vi "GetVIReference.vi"(5 "LVClassLibrary in":refnum<vi>, 6 "template (if new)":path, 7 "application reference":refnum<vi>, 8 "error in":errorcluster, 9 "not in class":bool, 10 "vi type":T1(ring), 11 "file path":path) -> (0 "error out":errorcluster, 3 "reference out":refnum<vi>)   [LabVIEW 2013, in "control module data interface generator.lvlib"]
doc: "This VI creates a new file or open the reference if the file already exists"
uses:
  control module data interface generator.lvlib
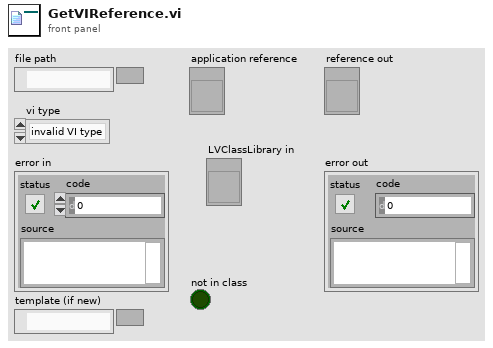
[diagram p1: front panel]
types:
  T1 = enum32{"invalid VI type", "Standard VI", "Control VI", "Global VI", "Polymorphic VI", "Configuration VI", "SubSystem", "Facade VI", "Method VI"}
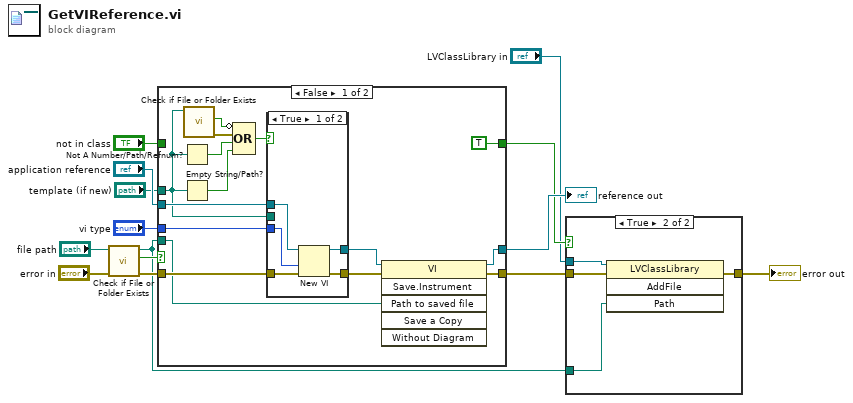
[diagram p0: block diagram]
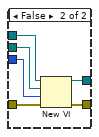
[diagram p3: hidden frame]
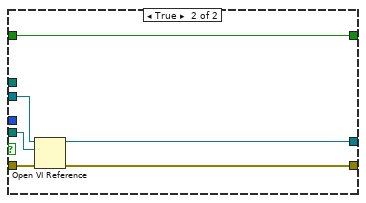
[diagram p4: hidden frame]
diagram:
  n1 = call <vilib>:"Check if File or Folder Exists.vi"("error in (no error)"="error in", "path"="file path") -> ("error out"=w12:errorcluster, "file or folder exists?"=w13:bool, "dup path"=w4:path)  [unwired: 7 in]
  n2 = case shown="False" w13 {
    tunnel: [w24 w44] -> w9
    tunnel: w12 -> [w29 w45]
    tunnel: w4 -> [w23 w46]
    tunnel: [w22 w43] -> w6
    tunnel: "vi type" -> [w27 _]
    tunnel: "application reference" -> [w26 w42]
    tunnel: [TRUE ("not in class") w41] -> w3
    tunnel: "not in class" -> [_ w41]
    tunnel: "template (if new)" -> [w16 _]
    frame False {
      n3 = Not A Number/Path/Refnum?(number/path/refnum=w16) -> (NaN/Path/Refnum?=w17:bool)
      n4 = Empty String/Path?(string/path=w16) -> (empty?=w18:bool)
      n5 = call <vilib>:"Check if File or Folder Exists.vi"("path"=w16) -> ("error out"=w20:errorcluster, "file or folder exists?"=w19:bool)  [unwired: 8 in, 1 out]
      n6 = Compound Arithmetic op=OR(invert w19, w20, w17, w18) -> (w15:bool)
      n7 = case shown="True" w15 {
        tunnel: w29 -> [w34 w40]
        tunnel: [w33 w39] -> w28
        tunnel: w27 -> [w32 w38]
        tunnel: w26 -> [w31 w37]
        tunnel: [w30 w36] -> w25
        tunnel: w16 -> [_ w35]
        frame True {
          n8 = New VI(8:w34, 9:w32, 11:w31) -> (0:w33:errorcluster, 3:w30:refnum<vi>)  [unwired: 4 out]
        }
        frame False {
          n9 = New VI(8:w40, 9:w38, 10:w35, 11:w37) -> (0:w39:errorcluster, 3:w36:refnum<vi>)  [unwired: 3 out]
        }
      }
      n10 = invoke class="VI" method="Save.Instrument"(reference=w25, error in=w28, "Path to saved file"=w23) -> (reference out=w24:refnum<vi>, error out=w22:errorcluster)  [unwired: 3 in, 4 out]
    }
    frame True {
      n11 = Open VI Reference(application reference (local)=w42, vi path=w46, error in (no error)=w45) -> (vi reference=w44:refnum<vi>, error out=w43:errorcluster)  [unwired: 3 in]
    }
  }
  "reference out" <- w9
  n12 = case shown="True" w3 {
    tunnel: w6 -> [w47 w51]
    tunnel: [w47 w50] -> w5
    tunnel: w4 -> [_ w49]
    tunnel: "LVClassLibrary in" -> [_ w48]
    frame False {
    }
    frame True {
      n13 = invoke class="LVClassLibrary" method="AddFile"(reference=w48, error in=w51, "Path"=w49) -> (error out=w50:errorcluster)  [unwired: 1 in, 3 out]
    }
  }
  "error out" <- w5
